vi "Kai.vi"() -> ()   [LabVIEW 2019]
uses:
  <vilib>/Instr/_visa.llb/VISA Configure Serial Port (Instr).vi
panel:
  in  "stop":bool
  out "str":string
  out "Vrms":dbl
  out "Hisory Waveform":dbl(graph)
  out "数值":dbl
  out "字符串":string
  in  "VISA resource name":refnum<visa-resource-name> caption="VISA资源名称"
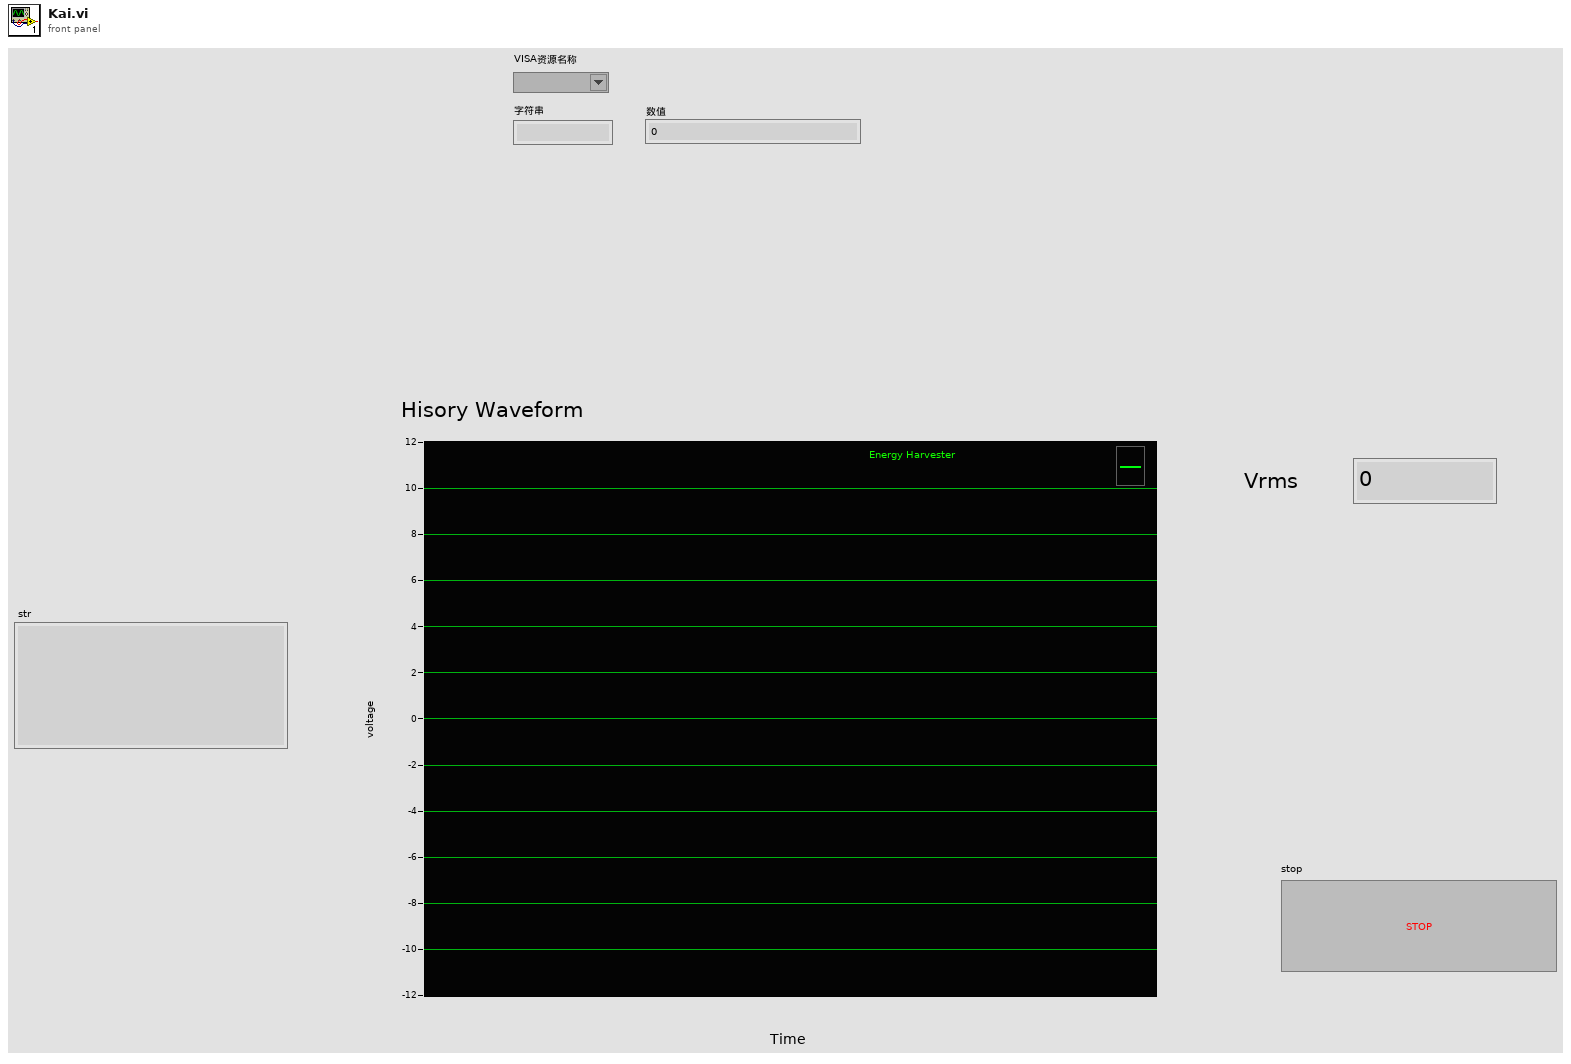
[diagram p1: front panel]
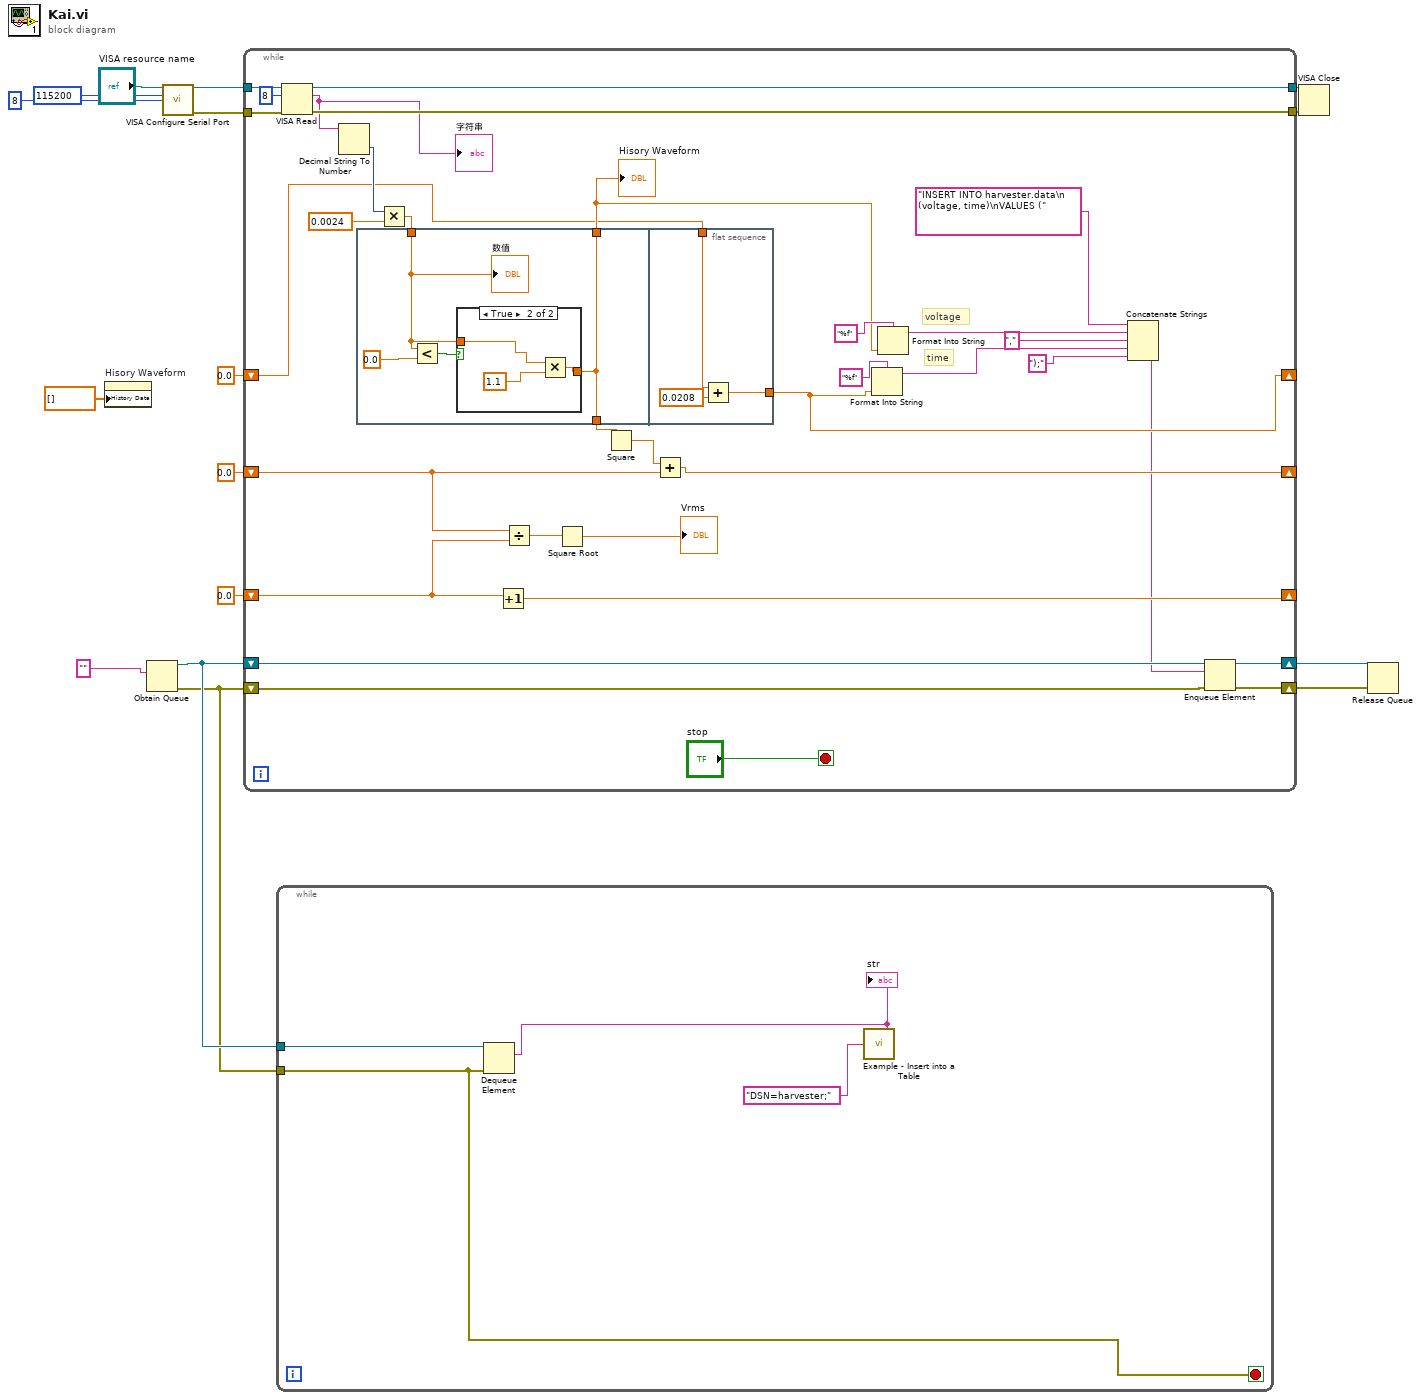
[diagram p0: block diagram]
diagram:
  n1 = property on="Hisory Waveform" class="WFChart (strict)"("History Data"=dbl[] []) -> ()  [unwired: 2 in, 2 out]
  n2 = Obtain Queue(element data type="" ("name (unnamed)")) -> (queue out=w3:refnum<queue>, error out=w2:errorcluster)  [unwired: 4 in, 1 out]
  n3 = call-poly "VISA Configure Serial Port"("VISA resource name"="VISA resource name", "baud rate (9600)"=u32 115200, "data bits (8)"=u16 8) -> ("VISA resource name out"=w16:refnum<visa-resource-name>, "error out"=w14:errorcluster)  [unwired: 11 in]
  n4 = while {
    tunnel: w16 -> [w49]
    tunnel: [w48] -> w15
    tunnel: w14 -> [w47]
    tunnel: [w46] -> w13
    shift-right: [w39] -> _
    shift-left: 0.0 -> [w37]
    shift-right: [w38] -> _
    shift-left: 0.0 -> [w36]
    shift-right: [w23] -> _
    shift-left: 0.0 -> [w24]
    shift-right: [w20] -> w5
    shift-left: w3 -> [w22]
    shift-right: [w19] -> w4
    shift-left: w2 -> [w21]
    stop <- "stop" stop-if-true
    # "time"
    # "voltage"
    n5 = VISA Read(VISA resource name=w49, byte count=u32 8 ("字节总数"), error in (no error)=w47) -> (VISA resource name out=w48:refnum<visa-resource-name>, read buffer=w44:string, error out=w46:errorcluster)  [unwired: 1 out]
    "字符串" <- w44
    n6 = Decimal String To Number(string=w44) -> (number=w42:i32)  [unwired: 2 in, 1 out]
    n7 = flat-sequence {
      tunnel: w41 -> [w51]
      tunnel: [w50] -> w25
      tunnel: [w50] -> w26
      tunnel: w24 -> [w59]
      tunnel: [w58] -> w23
      frame #0 {
        n8 = Less?(x=w51, y=0.0) -> (x < y?=w52:bool)
        n9 = case shown="True" w52 {
          tunnel: w51 -> [w54 w55]
          tunnel: [w54 w56] -> w50
          frame False {
          }
          frame True {
            n10 = Multiply(x=w55, y=1.1) -> (x*y=w56:dbl)
          }
        }
        "数值" <- w51
      }
      frame #1 {
        n11 = Add(x=w59, y=0.0208) -> (x+y=w58:dbl)
      }
    }
    n12 = Multiply(x=w42, y=0.0024) -> (x*y=w41:dbl)
    n13 = Increment(x=w36) -> (x+1=w38:dbl)
    n14 = Divide(x=w37, y=w36) -> (x/y=w35:dbl)
    n15 = Square Root(x=w35) -> (sqrt(x)=→"Vrms":dbl)
    n16 = Square(x=w26) -> (x^2=w40:dbl)
    n17 = Add(x=w40, y=w37) -> (x+y=w39:dbl)
    n18 = Format Into String(format string="%f", w23) -> (resulting string=w33:string)  [unwired: 2 in, 1 out]
    n19 = Format Into String(format string="%f", w25) -> (resulting string=w32:string)  [unwired: 2 in, 1 out]
    n20 = Concatenate Strings("INSERT INTO harvester.data\n (voltage, time)\nVALUES (", w32, "," ("string"), w33, ");" ("string")) -> (w18:string)
    n21 = Enqueue Element(queue=w22, element=w18, error in (no error)=w21) -> (queue out=w20:refnum<queue>, error out=w19:errorcluster)  [unwired: 1 in, 1 out]
    "Hisory Waveform" <- w25
  }
  n22 = while {
    tunnel: w3 -> [w63]
    tunnel: w2 -> [w61]
    stop <- w61 stop-if-true
    n23 = Dequeue Element(queue=w63, error in (no error)=w61) -> (element=w62:string)  [unwired: 1 in, 3 out]
    "str" <- w62
    n24 = call "Example - Insert into a Table.vi"("Command Text"=w62, "ConnectionString"="DSN=harvester;" ("Command Text")) -> ()
  }
  n25 = VISA Close(VISA resource name=w15, error in (no error)=w13) -> ()  [unwired: 1 out]
  n26 = Release Queue(queue=w5, error in (no error)=w4) -> ()  [unwired: 1 in, 3 out]
